vi "SUB-module-문자배열을 문자열로 변환.vi"(1 "배열":string[](array[string])) -> (0 "문자열":string)   [LabVIEW 2015]
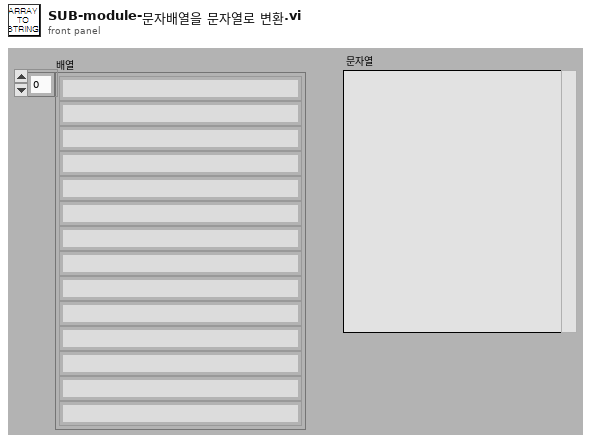
[diagram p1: front panel]
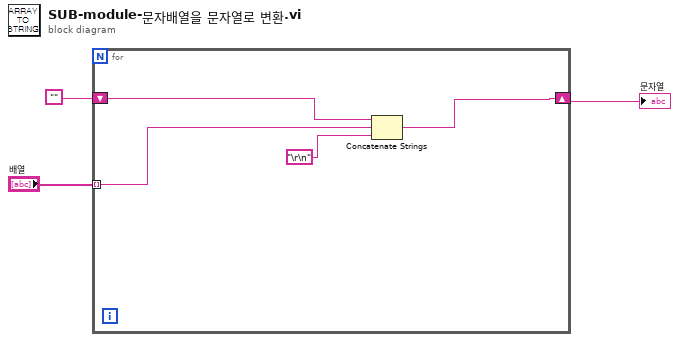
[diagram p0: block diagram]
diagram:
  n1 = for {
    shift-right: [w6] -> w1
    shift-left: "" -> [w7]
    tunnel: "배열" -> [w5] mode=indexing
    n2 = Concatenate Strings(w7, w5, "\r\n") -> (w6:string)
  }
  "문자열" <- w1
